vi "G1G2Converter_Installer.vi"() -> ()   [LabVIEW 2009]
panel:
  in  "Uninstall":bool
  out "Info":string
  in  "Cancel":bool
  out "License":string="G1G2 Converter\n\nCopyright (c) 2010, AddQ Consulting <http://www.addq.se>\n\nAll rights reserved."
  in  "Install":bool
  # "G1G2 Converter Installer"
  # "1. Installs G1G2 Converter in vi.lib/project."
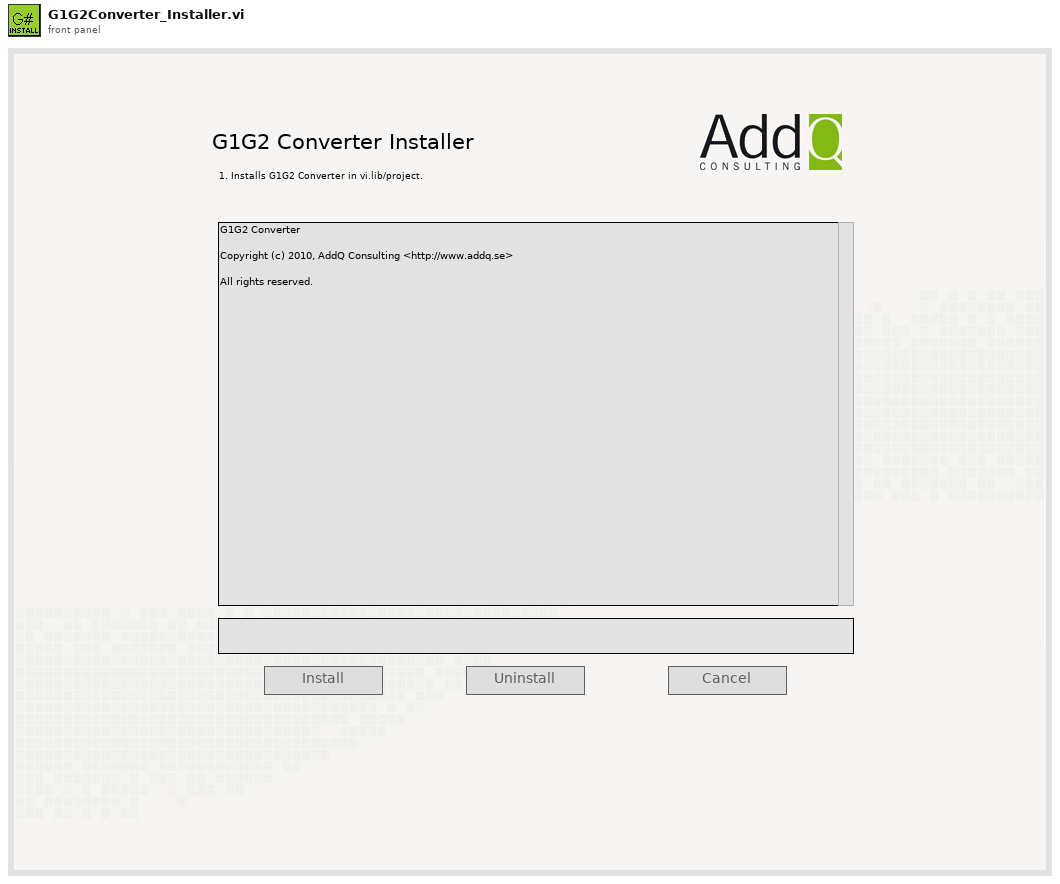
[diagram p1: front panel]
types:
  T1 = enum8{"Enabled", "Disabled", "Disabled and Grayed Out"}
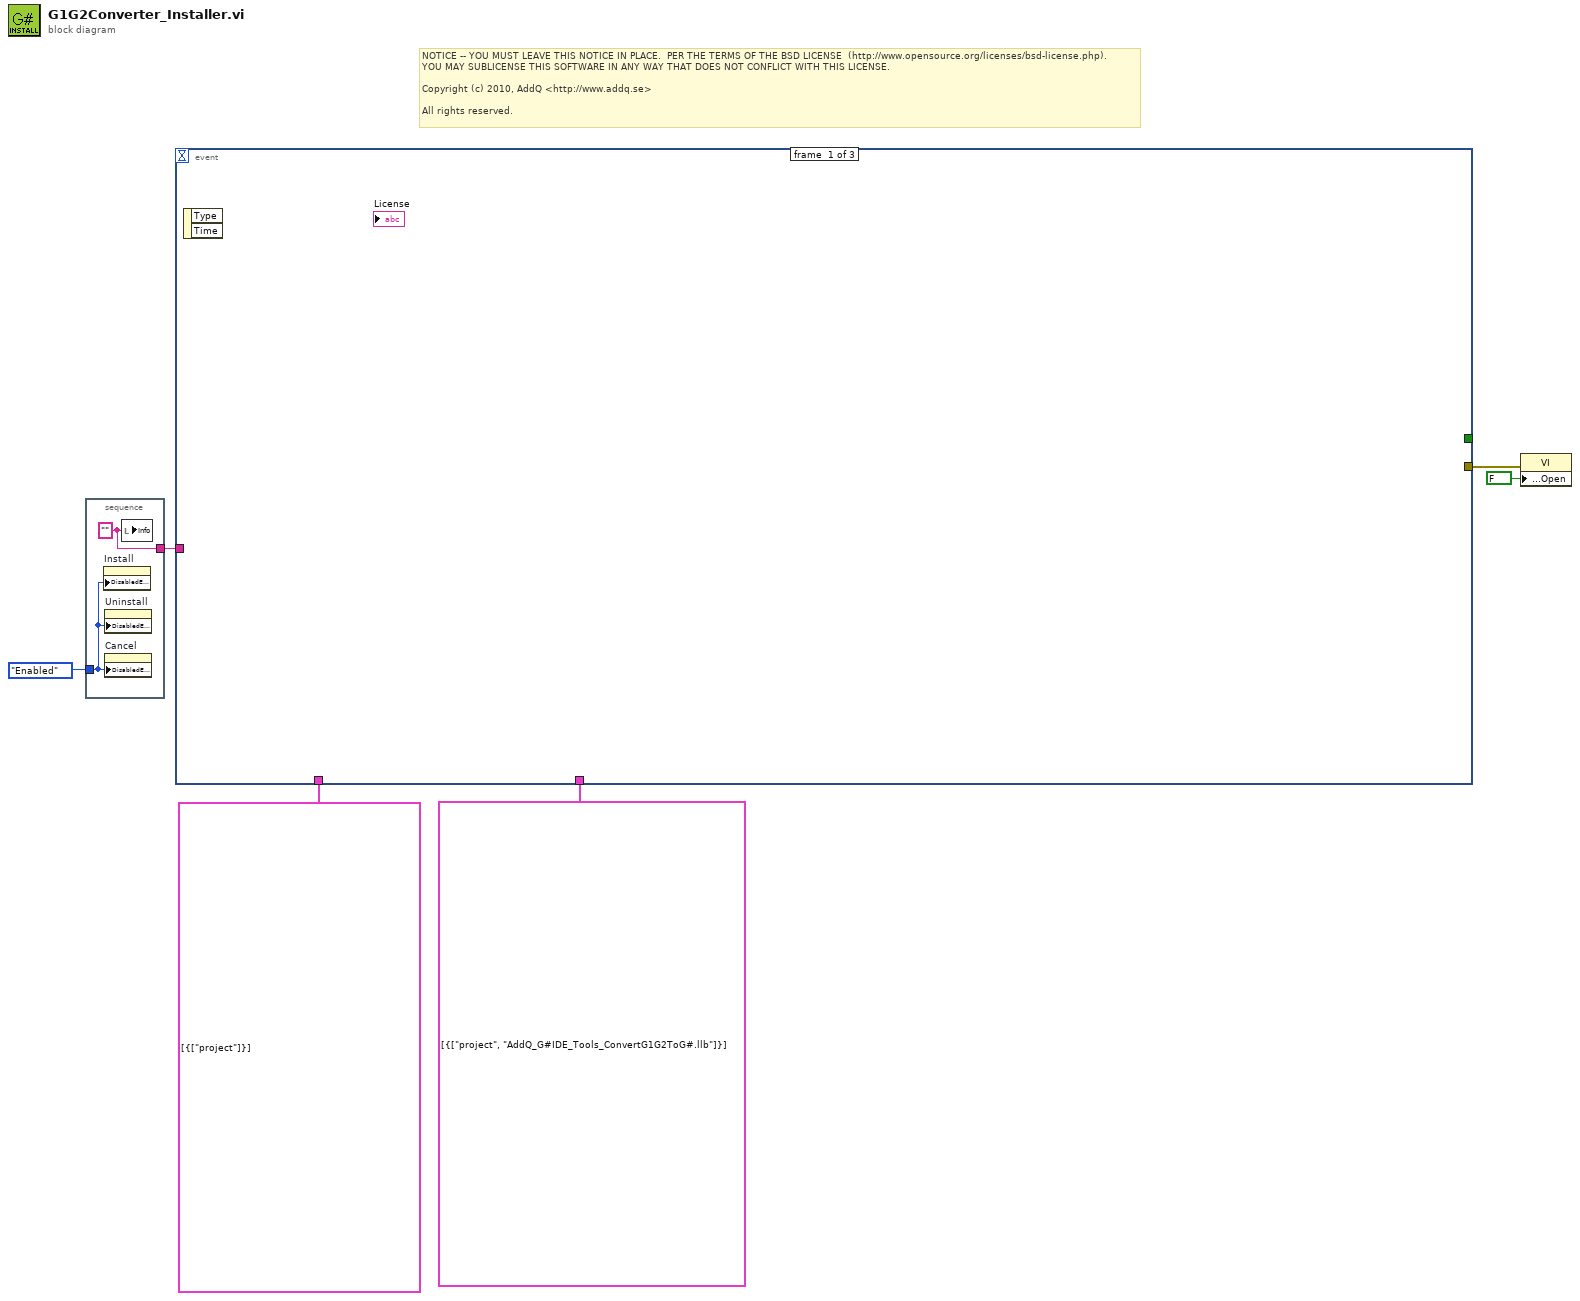
[diagram p0: block diagram]
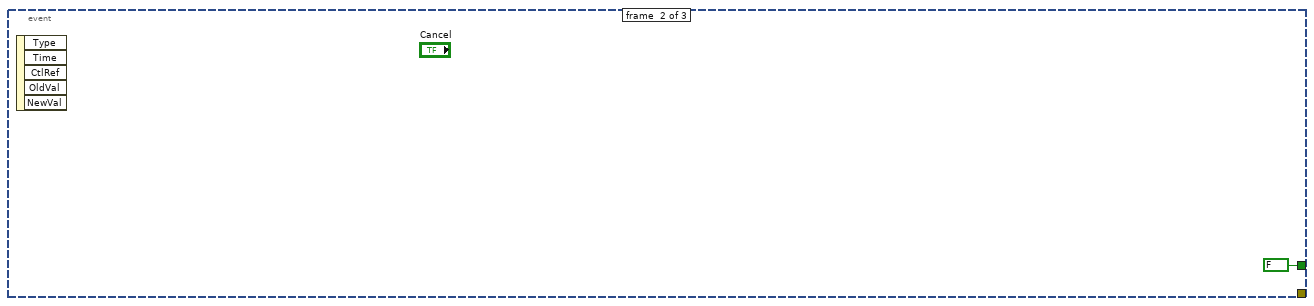
[diagram p2: hidden frame]
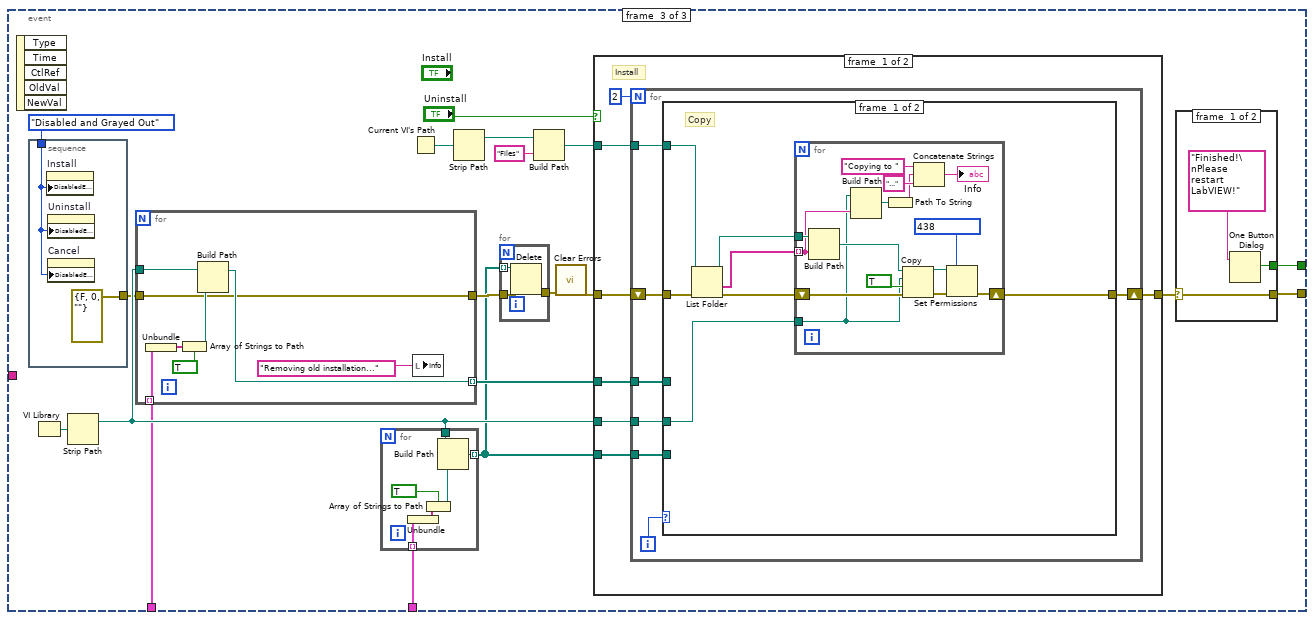
[diagram p3: hidden frame]
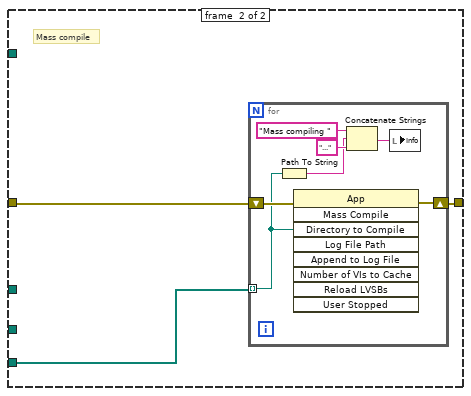
[diagram p4: hidden frame]
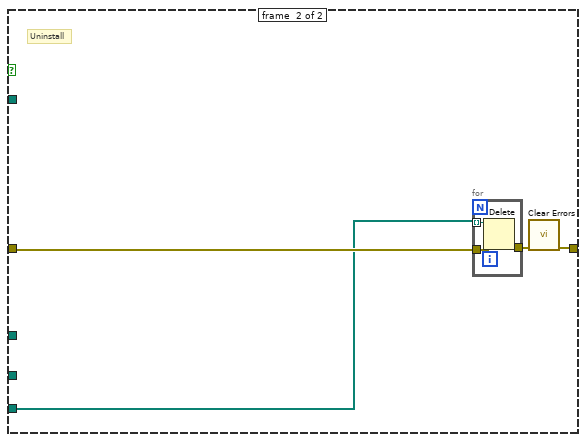
[diagram p5: hidden frame]
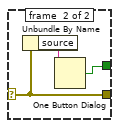
[diagram p6: hidden frame]
diagram:
  # "NOTICE -- YOU MUST LEAVE THIS NOTICE IN PLACE.  PER THE TERMS OF THE BSD LICENSE  (http://www.opensource.org/licenses/bsd-license.php).\nYOU MAY SUBLICENSE THIS SOFTWARE IN ANY WAY THAT DOES NOT CONFLICT WITH THIS LICENSE.\n\nCopyright (c) 2010, AddQ <http://www.addq.se>\n\nAll rights reserved."
  n1 = stacked-sequence {
    tunnel: [w8] -> w6
    tunnel: T1."Enabled" ("Disabled") -> [w7]
    frame #0 {
      w8 = "" ("Info")
      n2 = property on="Install" class="Bool"("DisabledEnum"=w7) -> ()  [unwired: 2 in, 2 out]
      n3 = property on="Uninstall" class="Bool"("DisabledEnum"=w7) -> ()  [unwired: 2 in, 2 out]
      n4 = property on="Cancel" class="Bool"("DisabledEnum"=w7) -> ()  [unwired: 2 in, 2 out]
      n5 = local write "Info"(w8) -> ()
    }
  }
  n6 = event shown="[2] \"Install\", \"Uninstall\": Value Change" {
    selector: _ -> [_ _ _]
    dyn-events: _ -> [_ _ _]
    timeout: _ -> [_ _ _]
    tunnel: w6 -> [_ _ _]
    tunnel: [_ _ w23] -> w5
    tunnel: cluster{string[]}[] [{["project"]}] -> [_ _ w12]
    tunnel: cluster{string[]}[] [{["project", "AddQ_G#IDE_Tools_ConvertG1G2ToG#.llb"]}] -> [_ _ w16]
    tunnel: [_ FALSE ("true") w11] -> _
    event #0 {
      n7 = event-data() -> ()  [unwired: 1 in, 2 out]
    }
    event #1 {
      n8 = event-data() -> ()  [unwired: 1 in, 5 out]
    }
    event #2 {
      n9 = event-data() -> ()  [unwired: 1 in, 5 out]
      n10 = stacked-sequence {
        tunnel: T1."Disabled and Grayed Out" ("Disabled") -> [w30]
        tunnel: [errorcluster {"status"=FALSE, "code"=0, "source"=""} ("error out")] -> w13
        frame #0 {
          n11 = property on="Install" class="Bool"("DisabledEnum"=w30) -> ()  [unwired: 2 in, 2 out]
          n12 = property on="Uninstall" class="Bool"("DisabledEnum"=w30) -> ()  [unwired: 2 in, 2 out]
          n13 = property on="Cancel" class="Bool"("DisabledEnum"=w30) -> ()  [unwired: 2 in, 2 out]
        }
      }
      n14 = VI Library() -> (path=w25:path)
      n15 = Strip Path(path=w25) -> (stripped path=w14:path)  [unwired: 1 out]
      n16 = for {
        tunnel: w14 -> [w100]
        tunnel: [w94] -> w17
        tunnel: [w95] -> w20 mode=indexing
        tunnel: w12 -> [w99] mode=indexing
        tunnel: w13 -> [w94]
        n17 = Unbundle(w99) -> (w98:string[])
        n18 = Array of Strings to Path(0:w98, 1:TRUE ("relative")) -> (2:w97:path)
        n19 = Build Path(base path=w100, name or relative path=w97) -> (appended path=w95:path)
        n20 = local write "Info"("Removing old installation..." ("string")) -> ()
      }
      n21 = for {
        tunnel: w14 -> [w36]
        tunnel: [w35] -> w10 mode=indexing
        tunnel: w16 -> [w34] mode=indexing
        n22 = Unbundle(w34) -> (w32:string[])
        n23 = Array of Strings to Path(0:w32, 1:TRUE ("relative")) -> (2:w31:path)
        n24 = Build Path(base path=w36, name or relative path=w31) -> (appended path=w35:path)
      }
      n25 = Current VI's Path() -> (path=w28:path)
      n26 = Strip Path(path=w28) -> (stripped path=w27:path)  [unwired: 1 out]
      n27 = for {
        tunnel: [w39] -> w18
        tunnel: w17 -> [w38]
        tunnel: w10 -> [w37] mode=indexing
        n28 = Delete(path (use dialog)=w37, error in=w38) -> (error out=w39:errorcluster)  [unwired: 3 in, 2 out]
      }
      n29 = Build Path(base path=w27, name or relative path="Files") -> (appended path=w24:path)
      n30 = call <vilib>:"Clear Errors.vi"("error in (no error)"=w18) -> ("error out"=w19:errorcluster)  [unwired: 6 in]
      n31 = case shown="False" "Uninstall" {
        tunnel: w24 -> [w46 _]
        tunnel: w14 -> [w45 _]
        tunnel: [w42 w88] -> w22
        tunnel: w20 -> [w41 _]
        tunnel: w19 -> [w44 w87]
        tunnel: w10 -> [w40 w86]
        frame #0 {
          # "Install"
          n32 = for {
            N: 2 -> [_]
            tunnel: w46 -> [w53]
            tunnel: w45 -> [w52]
            shift-right: [w50] -> w42
            shift-left: w44 -> [w51]
            tunnel: w41 -> [w48]
            tunnel: w40 -> [w47]
            i -> [w49]
            n33 = case shown="1" w49 {
              tunnel: w53 -> [w60 _]
              tunnel: w52 -> [w56 _]
              tunnel: w51 -> [w55 w77]
              tunnel: [w54 w78] -> w50
              tunnel: w48 -> [_ _]
              tunnel: w47 -> [_ w76]
              frame #0 {
                # "Copy"
                n34 = List Folder(path=w60, error in=w55) -> (path out=w58:path, folder names=w59:string[], error out=w57:errorcluster)  [unwired: 2 in, 1 out]
                n35 = for {
                  tunnel: w56 -> [w62]
                  tunnel: w59 -> [w63] mode=indexing
                  tunnel: w58 -> [w74]
                  shift-right: [w67] -> w54
                  shift-left: w57 -> [w71]
                  n36 = Build Path(base path=w74, name or relative path=w63) -> (appended path=w66:path)
                  n37 = Build Path(base path=w62, name or relative path=w63) -> (appended path=w64:path)
                  n38 = Path To String(path=w64) -> (string=w65:string)
                  n39 = Copy(8:w71, 9:TRUE ("overwrite (F)"), 10:w62, 11:w66) -> (0:w70:errorcluster, 3:w69:path)  [unwired: 1 in, 1 out]
                  n40 = Concatenate Strings("Copying to " ("string"), w65, "..." ("string")) -> (→"Info":string)
                  n41 = Set Permissions(7:i16 438 ("permissions"), 8:w70, 11:w69) -> (0:w67:errorcluster)  [unwired: 2 in, 1 out]
                }
              }
              frame #1 {
                # "Mass compile"
                n42 = for {
                  shift-right: [w84] -> w78
                  shift-left: w77 -> [w85]
                  tunnel: w76 -> [w80] mode=indexing
                  n43 = Path To String(path=w80) -> (string=w79:string)
                  n44 = invoke class="App" method="Mass Compile"(error in=w85, "Directory to Compile"=w80) -> (error out=w84:errorcluster)  [unwired: 7 in, 8 out]
                  n45 = Concatenate Strings("Mass compiling " ("string"), w79, "..." ("string")) -> (w81:string)
                  n46 = local write "Info"(w81) -> ()
                }
              }
            }
          }
        }
        frame #1 {
          # "Uninstall"
          n47 = for {
            tunnel: [w92] -> w89
            tunnel: w87 -> [w91]
            tunnel: w86 -> [w90] mode=indexing
            n48 = Delete(path (use dialog)=w90, error in=w91) -> (error out=w92:errorcluster)  [unwired: 3 in, 2 out]
          }
          n49 = call <vilib>:"Clear Errors.vi"("error in (no error)"=w89) -> ("error out"=w88:errorcluster)  [unwired: 6 in]
        }
      }
      n50 = case shown="No Error" w22 {
        selector: w22 -> [w103 w106]
        tunnel: [w103 w106] -> w23
        tunnel: [w101 w104] -> w11
        frame #0 {
          n51 = One Button Dialog(message="Finished!\nPlease restart LabVIEW!") -> (true=w101:bool)  [unwired: 1 in]
        }
        frame #1 {
          n52 = Unbundle By Name(w106) -> ("source"=w105:string)
          n53 = One Button Dialog(message=w105) -> (true=w104:bool)  [unwired: 1 in]
        }
      }
    }
  }
  n54 = property class="VI"(error in=w5, "Front Panel.Open"=FALSE ("Front Panel Window:Open")) -> ()  [unwired: 1 in, 2 out]
